vi "Plotmatrix Appearance Page.vi"() -> ()   [LabVIEW 2017, in "XY Plot Matrix.lvclass"]
uses:
  <vilib>/Math Plots/2D Math Plots/XY Plot Matrix/XY Plot Matrix/XY Plot Matrix.lvclass
  <vilib>/Math Plots/2D Math Plots/2D Plot/2D Plot/Typedef/Graph General Property.ctl
  <vilib>/Math Plots/2D Math Plots/2D Plot/Action String/XYPlotMatrix Ctrl Act Queue.ctl
  <vilib>/Math Plots/2D Math Plots/2D Plot/Action String/XYPlotMatrix Ctrl Act Cluster.ctl
  <vilib>/Math Plots/2D Math Plots/2D Plot/Action String/2DMathPlot State Class.ctl
  <vilib>/Math Plots/2D Math Plots/2D Plot/2D Plot/Typedef/Dialog State.ctl
  <vilib>/Math Plots/2D Math Plots/2D Plot/2D Plot/Typedef/Temp Graph Property Action.ctl
  <vilib>/Math Plots/2D Math Plots/2D Plot/2D Plot/Typedef/Temp Graph State.ctl
  <vilib>/Math Plots/2D Math Plots/2D Plot/2D Plot/2D Plot.lvclass
panel:
  in  "Event Registration":refnum<event-registration>
  in  "Control Ref Queue":T1
  out "Graph General Out":T2
  in  "Graph General In":T2
  in  "Legend:Plots Shown":u32=1 caption="Plots shown" min=1
  in  "Autosize Legend":bool caption="Auto size to plot names"
  in  "Legend:Visible":bool caption="Show plot legend"
  in  "Palette:Visible":bool caption="Show graph palette"
  in  "Height":u32 step=1
  in  "Width":u32 step=1
  in  "Enabled State":T3(radio)
  in  "Caption.Visible":bool caption="Caption"
  in  "Caption.Text":string caption="Caption Text"
  in  "Label.Text":string caption="Label Text"
  in  "Label.Visible":bool caption="Label"
  # "Caption"
  # "Label"
  # "Enabled State"
  # "Size"
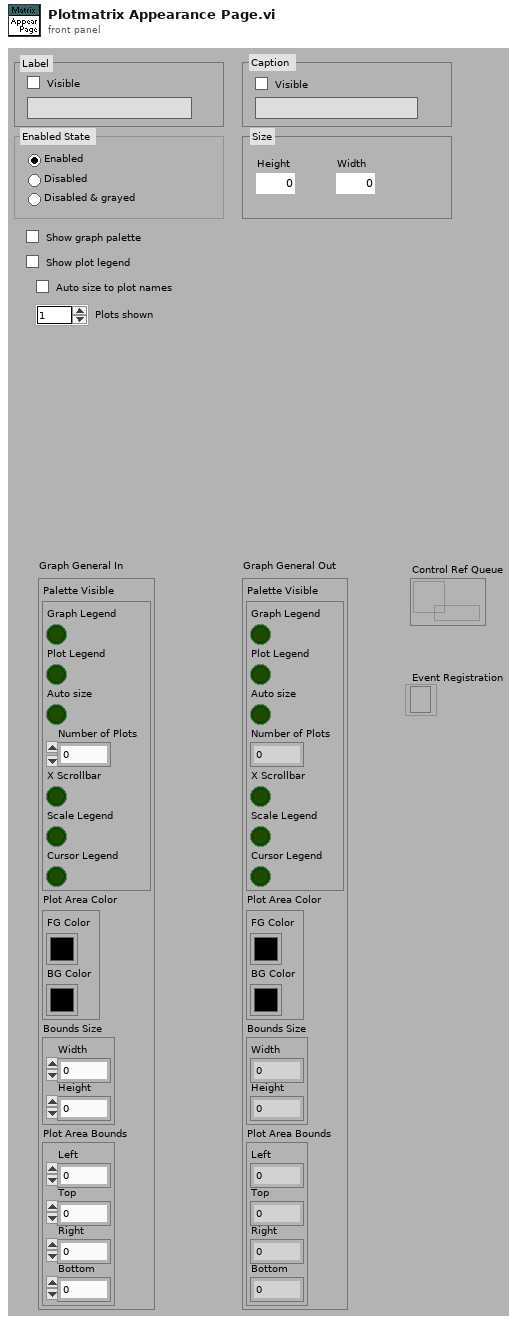
[diagram p1: front panel]
types:
  T1 = typedef "XYPlotMatrix Ctrl Act Queue.ctl" = refnum<queue>
  T2 = typedef "2D Plot.lvclass/Graph General Property.ctl" = cluster{"Palette Visible":cluster{"Graph Legend":bool, "Plot Legend":bool, "Auto size":bool, "Number of Plots":u32, "X Scrollbar":bool, "Scale Legend":bool, "Cursor Legend":bool}, "Plot Area Color":cluster{"FG Color":u32, "BG Color":u32}, "Bounds Size":cluster{"Width":u32, "Height":u32}, "Plot Area Bounds":cluster{"Left":i16, "Top":i16, "Right":i16, "Bottom":i16}}
  T3 = enum32{"Enabled", "Disabled", "Disabled & grayed", "Multiple Values"}
  T4 = typedef "2D Plot.lvclass/Dialog State.ctl" = enum16{"Initialize", "Read Property", "Write Property", "Idle", "Exit"}
  T5 = typedef "XYPlotMatrix Ctrl Act Cluster.ctl" = cluster{"Facade VI":refnum<vi>, "XControl":refnum<vi>, "Sub Panel":refnum<vi>, "Sub VI":refnum<vi>, "Export Image":refnum<vi>, "Display State Change Class":T6}
  T6 = typedef "2DMathPlot State Class.ctl" = enum16{"Update All (Undo)", "Update General", "Update Appearance", "Update Format", "Update Scale", "Update Marker", "Update Cursor", "None"}
  T7 = typedef "2D Plot.lvclass/Temp Graph State.ctl" = enum16{"Create", "Update Graph", "Update Property Only", "Get Plot Name", "Get Axis Name", "Destory"}
  T8 = typedef "2D Plot.lvclass/Temp Graph Property Action.ctl" = enum16{"Appearance Property", "Format Property", "Plots Property", "Scales Property"}
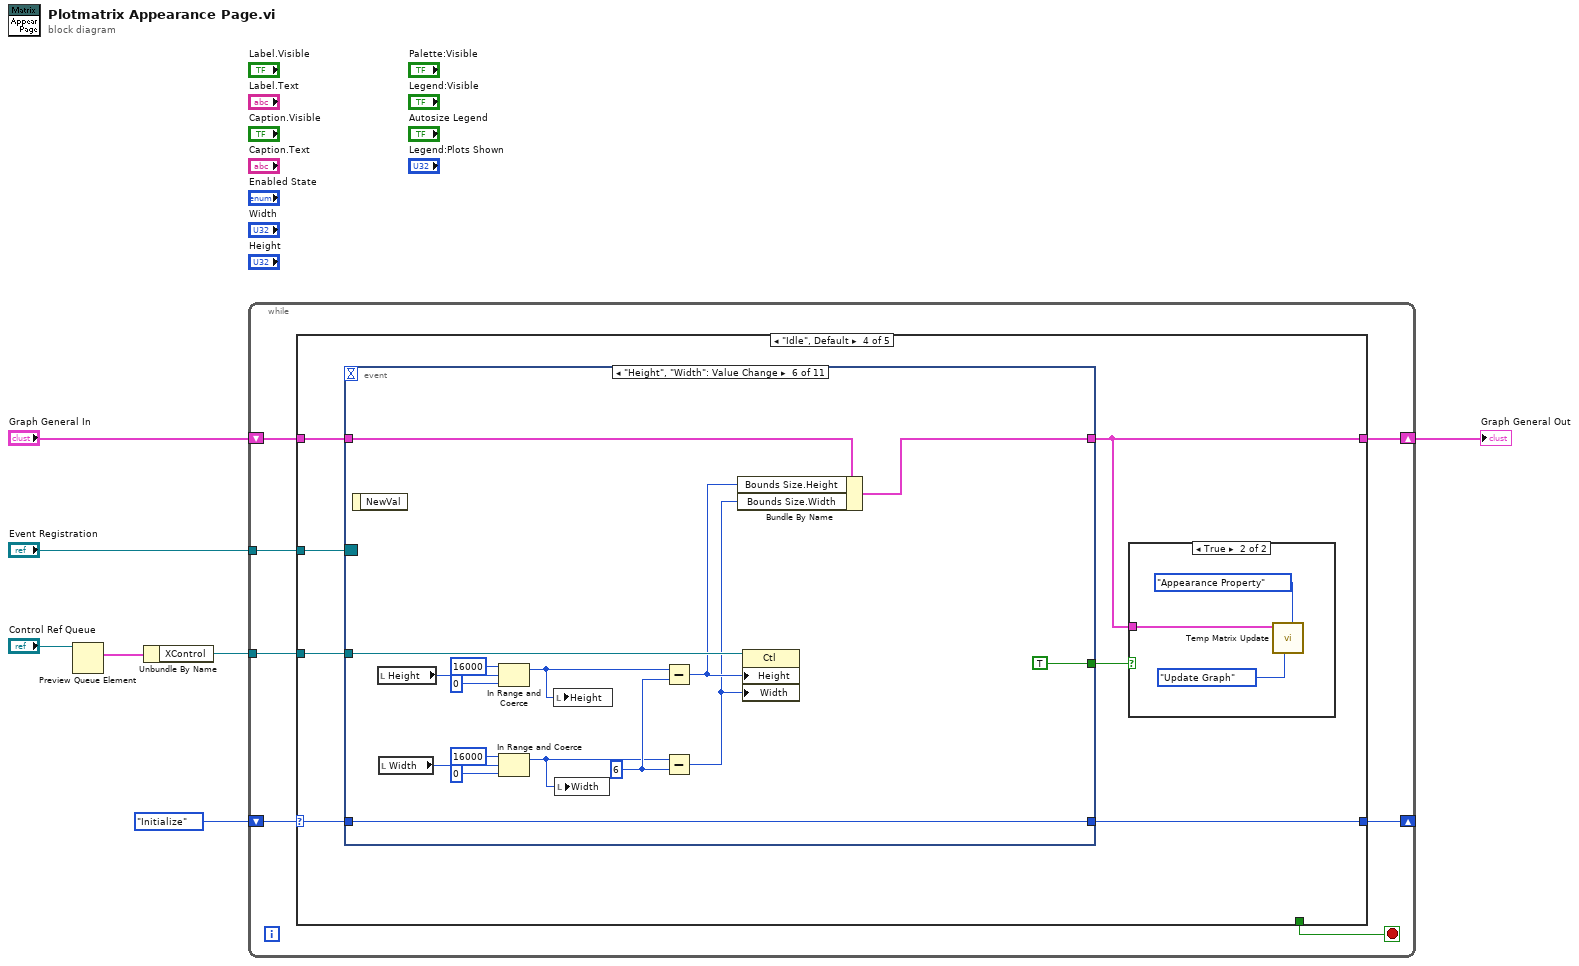
[diagram p0: block diagram]
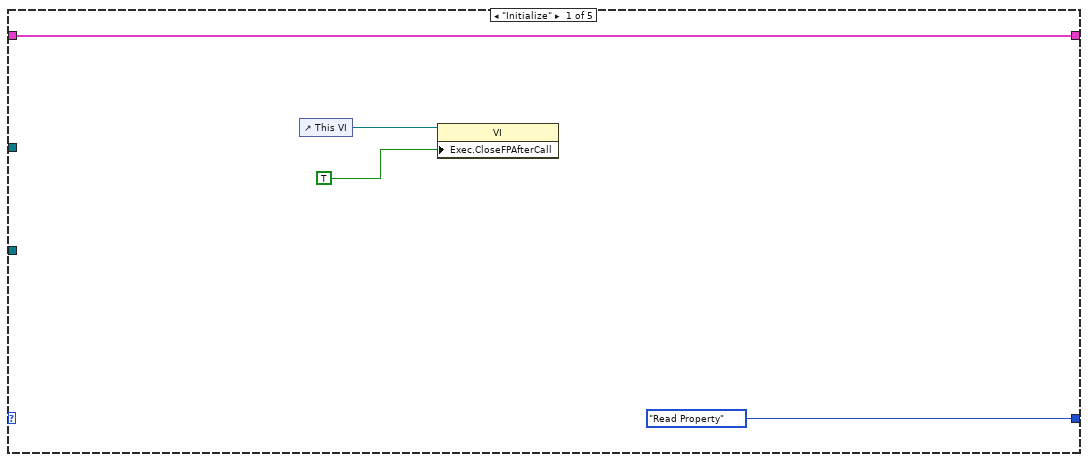
[diagram p2: hidden frame]
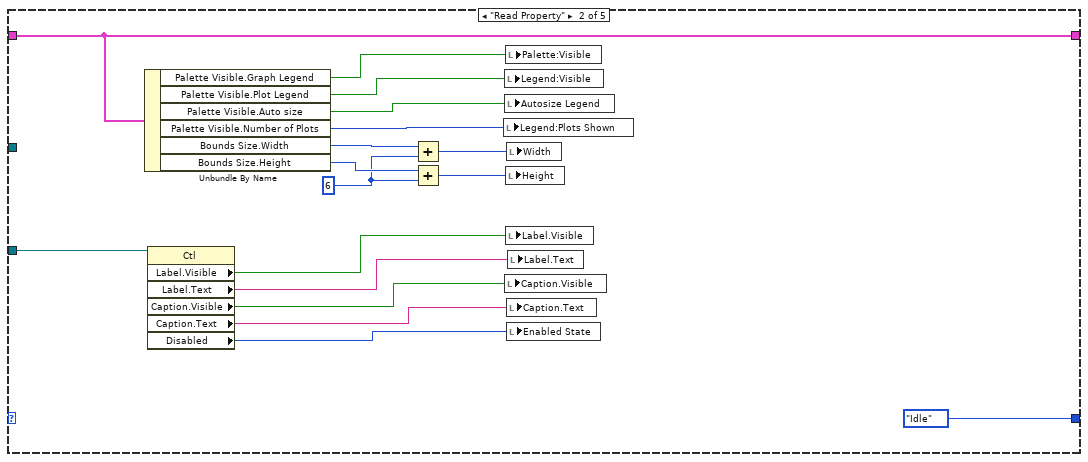
[diagram p3: hidden frame]
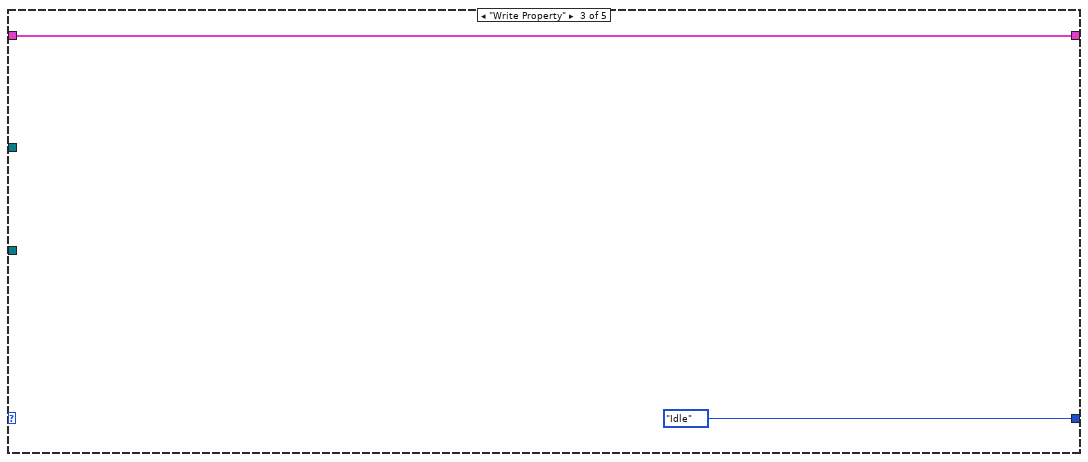
[diagram p4: hidden frame]
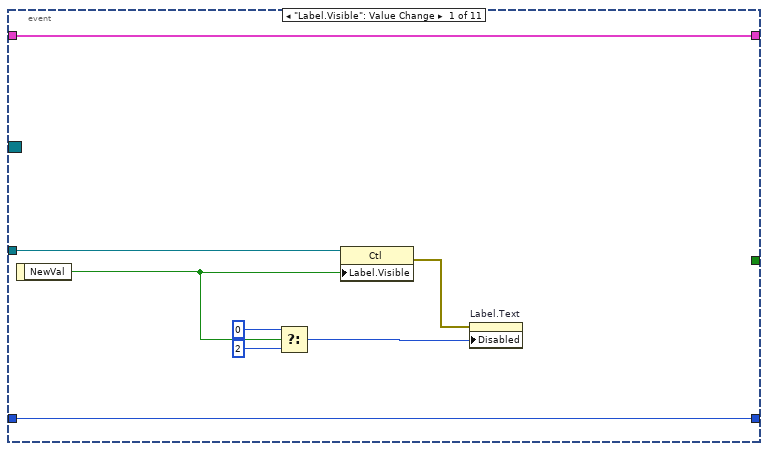
[diagram p6: hidden frame]
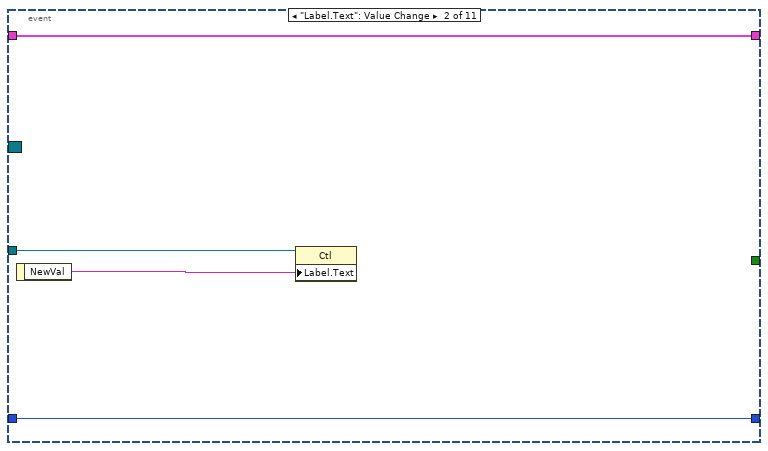
[diagram p7: hidden frame]
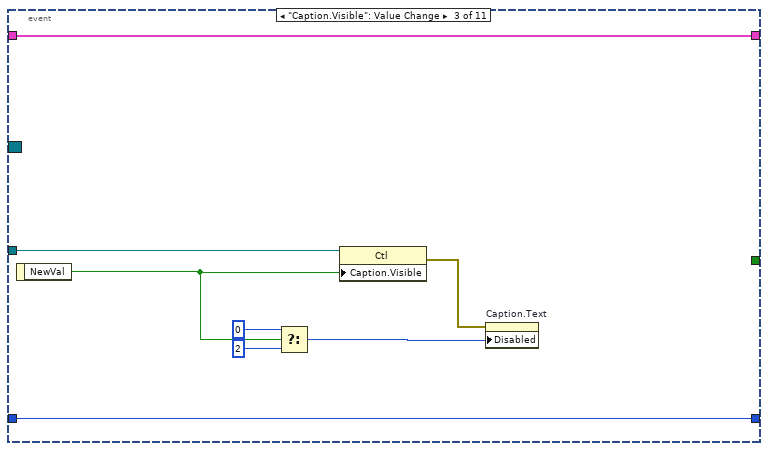
[diagram p8: hidden frame]
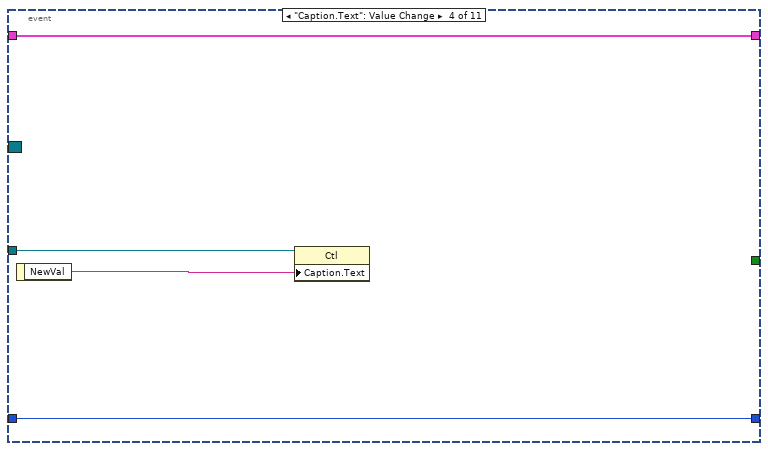
[diagram p9: hidden frame]
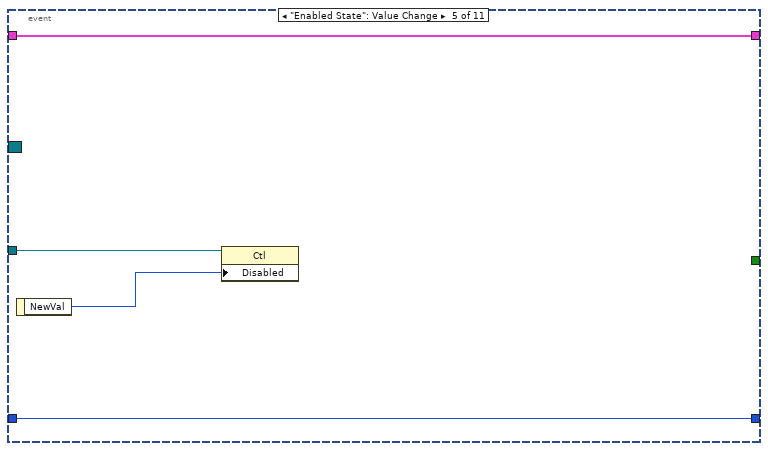
[diagram p10: hidden frame]
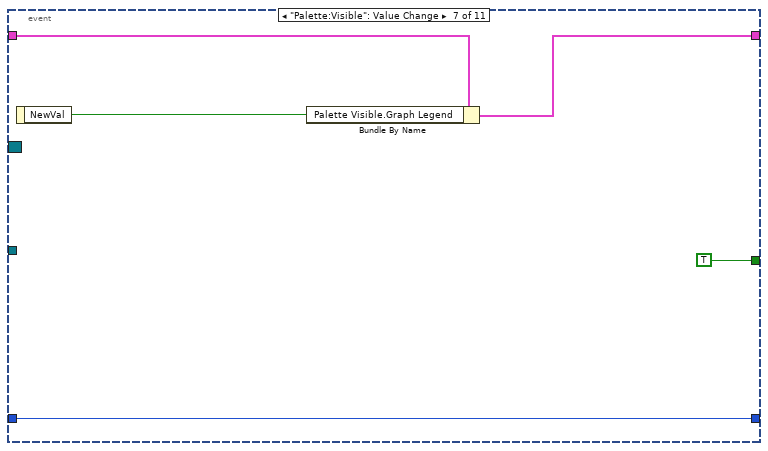
[diagram p11: hidden frame]
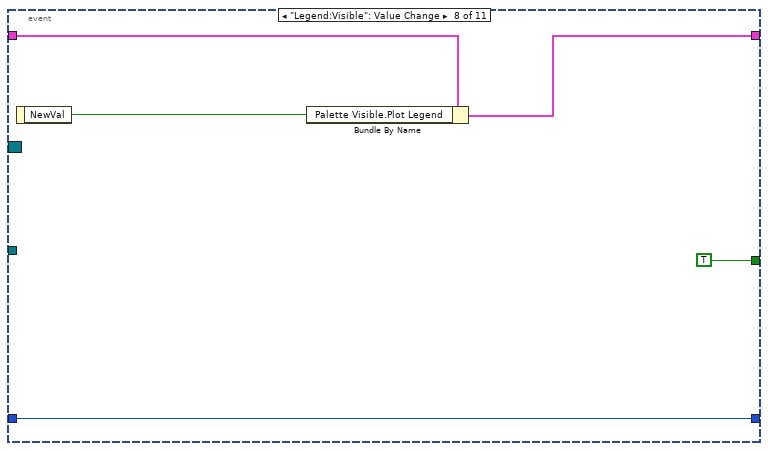
[diagram p12: hidden frame]
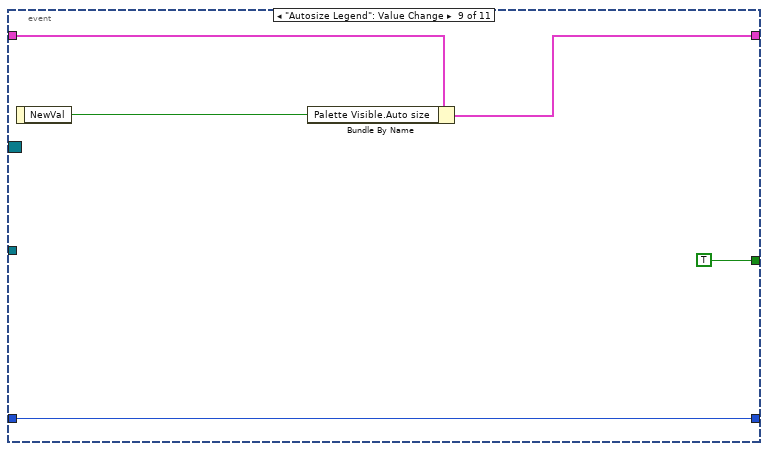
[diagram p13: hidden frame]
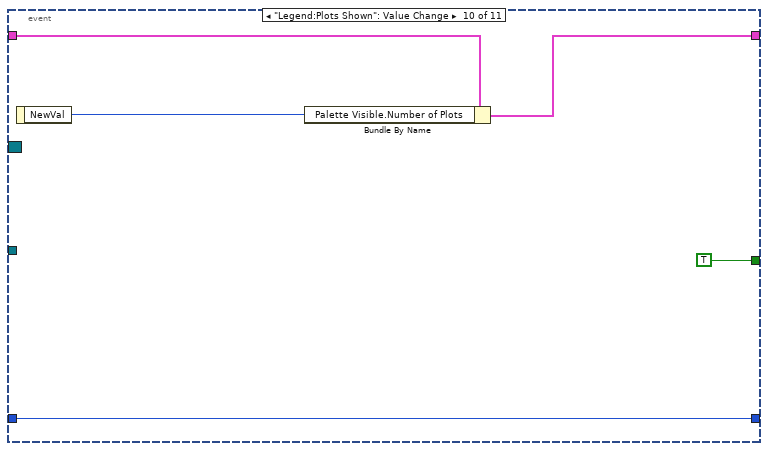
[diagram p14: hidden frame]
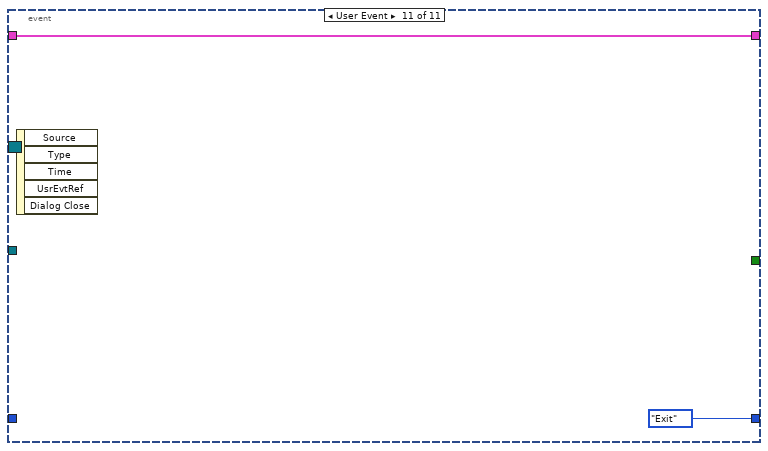
[diagram p15: hidden frame]
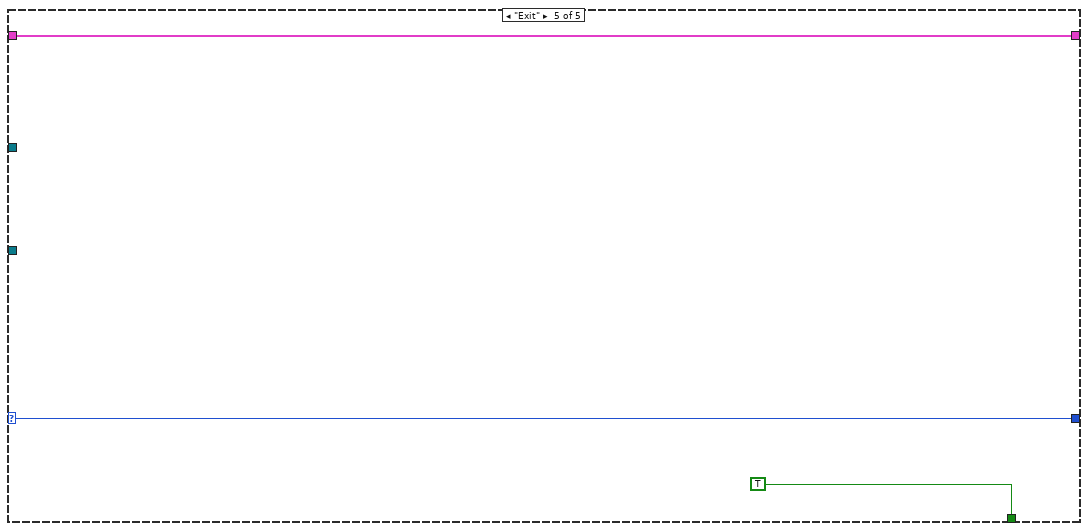
[diagram p16: hidden frame]
diagram:
  n1 = Preview Queue Element(queue="Control Ref Queue") -> (element=w1:T5)  [unwired: 1 in, 4 out]
  n2 = Unbundle By Name(w1) -> ("XControl"=w3:refnum<vi>)
  n3 = while {
    shift-right: [w12] -> _
    shift-left: Dialog_State."Initialize" ("Enum") -> [w14]
    shift-right: [w11] -> w6
    shift-left: "Graph General In" -> [w10]
    tunnel: w3 -> [w9]
    tunnel: "Event Registration" -> [w8]
    stop <- w13 stop-if-true
    n4 = case shown="\"Idle\", Default" w14 {
      selector: w14 -> [_ _ _ w40 w115]
      tunnel: [_ _ _ _ TRUE] -> w13
      tunnel: [Dialog_State."Read Property" ("Enum") Dialog_State."Idle" ("Enum") Dialog_State."Idle" ("Enum") w41 w115] -> w12
      tunnel: [w15 w24 w36 w38 w114] -> w11
      tunnel: w10 -> [w15 w24 w36 w44 w114]
      tunnel: w9 -> [_ w30 _ w43 _]
      tunnel: w8 -> [_ _ _ w42 _]
      frame "Initialize" {
        n5 = control-ref of="This VI"() -> (w17:refnum<vi>)
        n6 = property class="VI"(reference=w17, "Exec.CloseFPAfterCall"=TRUE ("Execution:Close After Call")) -> ()  [unwired: 1 in, 2 out]
      }
      frame "Read Property" {
        w19 = u32 6 ("y")
        n7 = Unbundle By Name(w24) -> ("Palette Visible.Graph Legend"=w34:bool, "Palette Visible.Plot Legend"=w33:bool, "Palette Visible.Auto size"=w32:bool, "Palette Visible.Number of Plots"=w31:u32, "Bounds Size.Width"=w23:u32, "Bounds Size.Height"=w22:u32)
        n8 = property class="Ctl"(reference=w30) -> ("Label.Visible"=w29:bool, "Label.Text"=w28:string, "Caption.Visible"=w27:bool, "Caption.Text"=w26:string, "Disabled"=w25:u8)  [unwired: 1 in, 2 out]
        n9 = Add(x=w23, y=w19) -> (x+y=w21:u32)
        n10 = Add(x=w22, y=w19) -> (x+y=w20:u32)
        n11 = local write "Legend:Plots Shown"(w31) -> ()
        n12 = local write "Legend:Visible"(w33) -> ()
        n13 = local write "Autosize Legend"(w32) -> ()
        n14 = local write "Caption.Visible"(w27) -> ()
        n15 = local write "Palette:Visible"(w34) -> ()
        n16 = local write "Height"(w20) -> ()
        n17 = local write "Label.Visible"(w29) -> ()
        n18 = local write "Width"(w21) -> ()
        n19 = local write "Caption.Text"(w26) -> ()
        n20 = local write "Enabled State"(w25) -> ()
        n21 = local write "Label.Text"(w28) -> ()
      }
      frame "Write Property" {
      }
      frame "Idle", Default {
        n22 = event shown="[5] \"Height\", \"Width\": Value Change" {
          selector: w42 -> [_ _ _ _ _ _ _ _ _ _ _]
          dyn-events: _ -> [_ _ _ _ _ _ _ _ _ _ _]
          timeout: _ -> [_ _ _ _ _ _ _ _ _ _ _]
          tunnel: w44 -> [w55 w57 w67 w69 w73 w91 w96 w101 w106 w111 w113]
          tunnel: [w55 w57 w67 w69 w73 w89 w95 w100 w105 w110 w113] -> w38
          tunnel: w43 -> [w54 w59 w66 w71 w75 w87 _ _ _ _ _]
          tunnel: [w48 w56 w60 w68 w72 w90 w93 w98 w103 w108 Dialog_State."Exit" ("Enum")] -> w41
          tunnel: w40 -> [w48 w56 w60 w68 w72 w90 w93 w98 w103 w108 _]
          tunnel: [_ _ _ _ _ TRUE TRUE TRUE TRUE TRUE _] -> w39
          event "Label.Visible": Value Change {
            n23 = event-data() -> ("NewVal"=w53:bool)  [unwired: 1 out]
            n24 = Select(t=u8 0 ("Disabled"), s=w53, f=u8 2 ("Disabled")) -> (s? t:f=w50:u8)
            n25 = property class="Ctl"(reference=w54, "Label.Visible"=w53) -> (error out=w49:errorcluster)  [unwired: 1 in, 1 out]
            n26 = property on="Label.Text" class="Str"(error in=w49, "Disabled"=w50) -> ()  [unwired: 1 in, 2 out]
          }
          event "Label.Text": Value Change {
            n27 = event-data() -> ("NewVal"=w58:string)  [unwired: 1 out]
            n28 = property class="Ctl"(reference=w59, "Label.Text"=w58) -> ()  [unwired: 1 in, 2 out]
          }
          event "Caption.Visible": Value Change {
            n29 = event-data() -> ("NewVal"=w65:bool)  [unwired: 1 out]
            n30 = Select(t=u8 0 ("Disabled"), s=w65, f=u8 2 ("Disabled")) -> (s? t:f=w62:u8)
            n31 = property class="Ctl"(reference=w66, "Caption.Visible"=w65) -> (error out=w61:errorcluster)  [unwired: 1 in, 1 out]
            n32 = property on="Caption.Text" class="Str"(error in=w61, "Disabled"=w62) -> ()  [unwired: 1 in, 2 out]
          }
          event "Caption.Text": Value Change {
            n33 = event-data() -> ("NewVal"=w70:string)  [unwired: 1 out]
            n34 = property class="Ctl"(reference=w71, "Caption.Text"=w70) -> ()  [unwired: 1 in, 2 out]
          }
          event "Enabled State": Value Change {
            n35 = event-data() -> ("NewVal"=w74:T3)  [unwired: 1 out]
            n36 = property class="Ctl"(reference=w75, "Disabled"=w74) -> ()  [unwired: 1 in, 2 out]
          }
          event "Height", "Width": Value Change {
            w84 = u32 6 ("x")
            n37 = event-data() -> ()  [unwired: 2 out]
            n38 = local read "Height"() -> (w79:u32)
            n39 = local read "Width"() -> (w78:u32)
            n40 = In Range and Coerce(upper limit=u32 16000, x=w79, lower limit=u32 0) -> (coerced(x)=w76:u32)  [unwired: 1 out]
            n41 = In Range and Coerce(upper limit=u32 16000, x=w78, lower limit=u32 0) -> (coerced(x)=w77:u32)  [unwired: 1 out]
            n42 = local write "Height"(w76) -> ()
            n43 = local write "Width"(w77) -> ()
            n44 = Subtract(x=w76, y=w84) -> (x-y=w86:u32)
            n45 = Subtract(x=w77, y=w84) -> (x-y=w85:u32)
            n46 = Bundle By Name(cluster=w91, "Bounds Size.Height"=w86, "Bounds Size.Width"=w85) -> (w89:T2)
            n47 = property class="Ctl"(reference=w87, "Height"=w86, "Width"=w85) -> ()  [unwired: 1 in, 2 out]
          }
          event "Palette:Visible": Value Change {
            n48 = event-data() -> ("NewVal"=w94:bool)  [unwired: 1 out]
            n49 = Bundle By Name(cluster=w96, "Palette Visible.Graph Legend"=w94) -> (w95:T2)
          }
          event "Legend:Visible": Value Change {
            n50 = event-data() -> ("NewVal"=w99:bool)  [unwired: 1 out]
            n51 = Bundle By Name(cluster=w101, "Palette Visible.Plot Legend"=w99) -> (w100:T2)
          }
          event "Autosize Legend": Value Change {
            n52 = event-data() -> ("NewVal"=w104:bool)  [unwired: 1 out]
            n53 = Bundle By Name(cluster=w106, "Palette Visible.Auto size"=w104) -> (w105:T2)
          }
          event "Legend:Plots Shown": Value Change {
            n54 = event-data() -> ("NewVal"=w109:u32)  [unwired: 1 out]
            n55 = Bundle By Name(cluster=w111, "Palette Visible.Number of Plots"=w109) -> (w110:T2)
          }
          event User Event {
            n56 = event-data() -> ()  [unwired: 6 out]
          }
        }
        n57 = case shown="True" w39 {
          tunnel: w38 -> [_ w47]
          frame False {
          }
          frame True {
            n58 = call <vilib>:"Temp Matrix Update.vi"("Property Name"=Temp_Graph_Property_Action."Appearance Property", "State"=Temp_Graph_State."Update Graph", "Property In"=w47) -> ()  [unwired: 2 in, 7 out]
          }
        }
      }
      frame "Exit" {
      }
    }
  }
  "Graph General Out" <- w6
